vi "rqcBob Modulator (FPGA).vi"(0 "rqcBob HW Control in":T1, 1 "clock in":bool, 2 "reset":bool, 12 "mod.clock delay":fxp<+,4,4>) -> (4 "rqcBob HW Control out":T1)   [LabVIEW 2018]
uses:
  Custom Controls/rqcBob HW Control.ctl
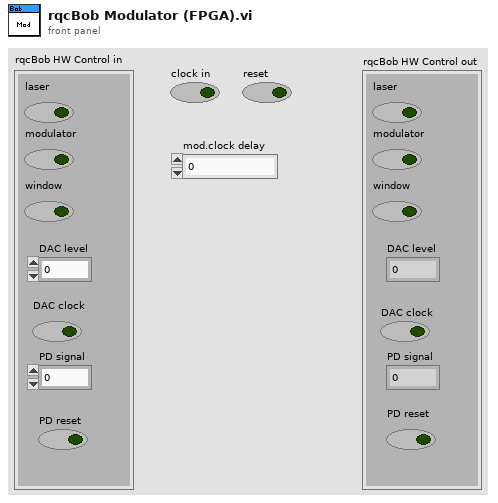
[diagram p1: front panel]
types:
  T1 = typedef "rqcBob HW Control.ctl" = cluster{"laser":bool, "modulator":bool, "window":bool, "DAC level":u8, "DAC clock":bool, "PD signal":u8, "PD reset":bool}
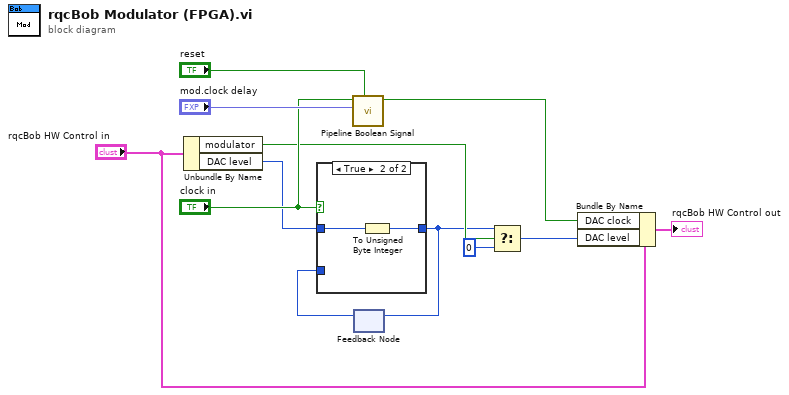
[diagram p0: block diagram]
diagram:
  n1 = Unbundle By Name("rqcBob HW Control in") -> ("modulator"=w7:bool, "DAC level"=w6:u8)
  n2 = call <vilib>:"Pipeline Boolean Signal.vi"("reset"="reset", "delay"="mod.clock delay", "input signal"="clock in") -> ("output signal"=w5:bool)  [unwired: 8 in]
  n3 = feedback #1() -> (w11:u8)  [unwired: 1 in]
  n4 = case shown="True" "clock in" {
    tunnel: [w13 w15] -> w2
    tunnel: w11 -> [w13 _]
    tunnel: w6 -> [_ w14]
    frame False {
    }
    frame True {
      n5 = To Unsigned Byte Integer(number=w14) -> (unsigned 8bit integer=w15:u8)
    }
  }
  n6 = feedback-in #1(w2) -> ()
  n7 = Select(t=w2, s=w7, f=u8 0) -> (s? t:f=w1:u8)
  n8 = Bundle By Name(cluster="rqcBob HW Control in", "DAC clock"=w5, "DAC level"=w1) -> (→"rqcBob HW Control out":T1)
